vi "Boiler room teest 2.vi"() -> ()   [LabVIEW 2023]
uses:
  Heater.vi
  AC.vi
panel:
  out "temp":dbl
  in  "?":dbl(knob) min=0.0 max=2.0 step=1.0 scale=0.0..2.0
  in  "stop":bool
  out "Thermometer":dbl(slide) scale=0.0..100.0
  in  "min temp":dbl=20.0
  in  "max temp":dbl=80.0
  in  "Automatic / Manual":bool
  out "AC":bool
  out "Heater":bool
  # "Heater"
  # "OFF"
  # "AC"
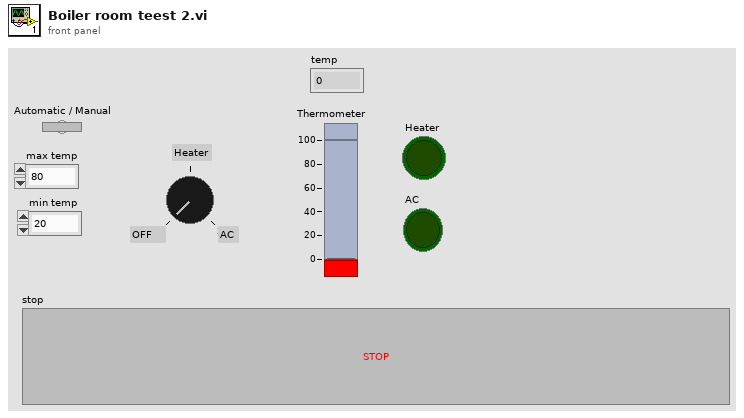
[diagram p1: front panel]
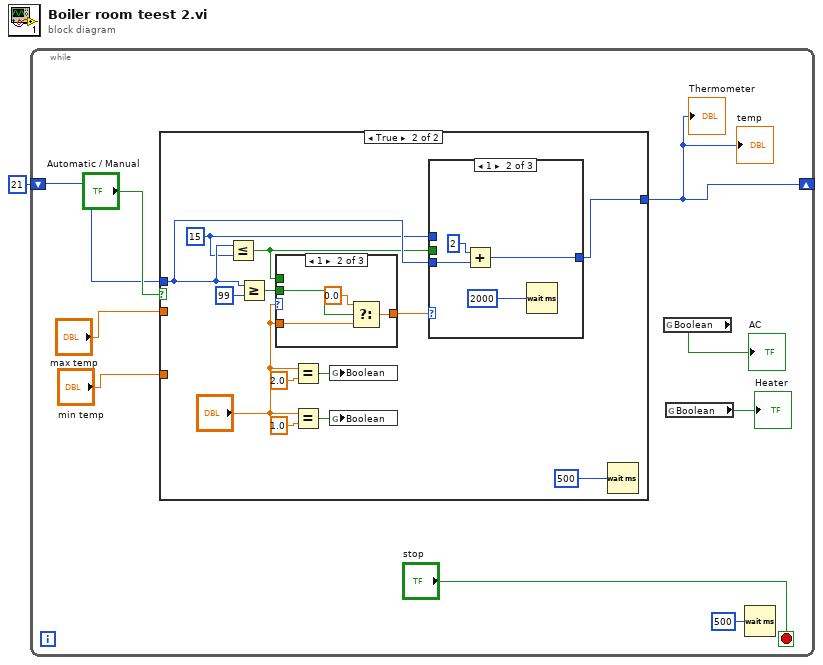
[diagram p0: block diagram]
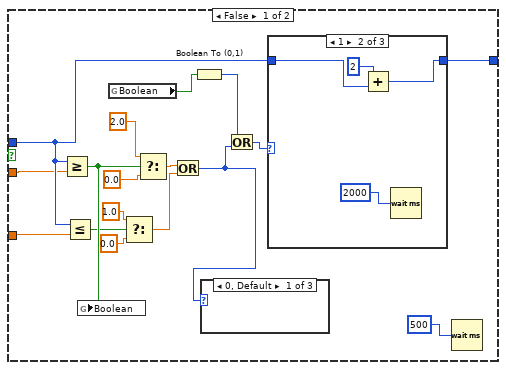
[diagram p2: hidden frame]
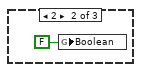
[diagram p3: hidden frame]
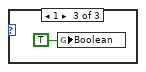
[diagram p4: hidden frame]
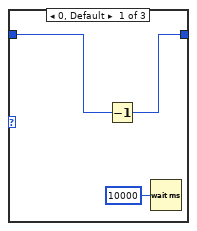
[diagram p5: hidden frame]
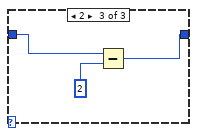
[diagram p6: hidden frame]
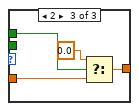
[diagram p8: hidden frame]
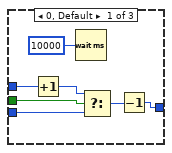
[diagram p9: hidden frame]
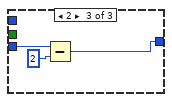
[diagram p10: hidden frame]
diagram:
  n1 = while {
    shift-right: [w5] -> _
    shift-left: 21 -> [w2]
    stop <- "stop" stop-if-true
    n2 = case shown="True" "Automatic / Manual" {
      tunnel: w2 -> [w20 w45]
      tunnel: "max temp" -> [w19 _]
      tunnel: "min temp" -> [w18 _]
      tunnel: [w22 w51] -> w5
      frame False {
        n3 = Greater Or Equal?(x=w20, y=w19) -> (x >= y?=w16:bool)
        n4 = Less Or Equal?(x=w20, y=w18) -> (x <= y?=w15:bool)
        n5 = global write "AC.vi" "Boolean"(w16) -> ()
        n6 = global read "Heater.vi" "Boolean"() -> (w11:bool)
        n7 = Select(t=1.0, s=w15, f=0.0) -> (s? t:f=w17:dbl)
        n8 = Select(t=2.0, s=w16, f=0.0) -> (s? t:f=w23:dbl)
        n9 = Or(x=w23, y=w17) -> (x .or. y?=w14:i32)
        n10 = Boolean To (0,1)(Boolean=w11) -> (0, 1=w12:i16)
        n11 = case shown="0, Default" w14 {
          frame 0, Default {
          }
          frame 2 {
            n12 = global write "Heater.vi" "Boolean"(FALSE ("Boolean")) -> ()
          }
          frame 1 {
            n13 = global write "Heater.vi" "Boolean"(TRUE ("Boolean")) -> ()
          }
        }
        n14 = Or(x=w12, y=w14) -> (x .or. y?=w13:i32)
        n15 = case shown="1" w13 {
          tunnel: w20 -> [w32 w36 w39]
          tunnel: [w31 w34 w38] -> w22
          frame 0, Default {
            n16 = Decrement(x=w32) -> (x-1=w31:i32)
            n17 = Wait (ms)(milliseconds to wait=u32 10000) -> ()  [unwired: 1 out]
          }
          frame 1 {
            n18 = Add(x=2, y=w36) -> (x+y=w34:i32)
            n19 = Wait (ms)(milliseconds to wait=u32 2000) -> ()  [unwired: 1 out]
          }
          frame 2 {
            n20 = Subtract(x=w39, y=2) -> (x-y=w38:i32)
          }
        }
        n21 = Wait (ms)(milliseconds to wait=u32 500) -> ()  [unwired: 1 out]
      }
      frame True {
        w40 = 15
        n22 = Less Or Equal?(x=w45, y=w40) -> (x <= y?=w41:bool)
        n23 = Greater Or Equal?(x=w45, y=99 ("x")) -> (x >= y?=w42:bool)
        n24 = case shown="1" "?" {
          tunnel: "?" -> [w53 w54 w59]
          tunnel: [w53 w56 w60] -> w50
          tunnel: w42 -> [_ w57 _]
          tunnel: w41 -> [_ _ w61]
          frame 0, Default {
          }
          frame 1 {
            n25 = Select(t=0.0 ("f"), s=w57, f=w54) -> (s? t:f=w56:dbl)
          }
          frame 2 {
            n26 = Select(t=0.0, s=w61, f=w59) -> (s? t:f=w60:dbl)
          }
        }
        n27 = Equal?(x="?", y=2.0) -> (x = y?=w46:bool)
        n28 = Equal?(x="?", y=1.0) -> (x = y?=w48:bool)
        n29 = global write "AC.vi" "Boolean"(w46) -> ()
        n30 = global write "Heater.vi" "Boolean"(w48) -> ()
        n31 = case shown="1" w50 {
          tunnel: w45 -> [w65 w72 w75]
          tunnel: [w68 w71 w74] -> w51
          tunnel: w41 -> [w66 _ _]
          tunnel: w40 -> [w63 _ _]
          frame 0, Default {
            n32 = Increment(x=w63) -> (x+1=w62:i32)
            n33 = Wait (ms)(milliseconds to wait=u32 10000) -> ()  [unwired: 1 out]
            n34 = Select(t=w62, s=w66, f=w65) -> (s? t:f=w64:i32)
            n35 = Decrement(x=w64) -> (x-1=w68:i32)
          }
          frame 1 {
            n36 = Add(x=2, y=w72) -> (x+y=w71:i32)
            n37 = Wait (ms)(milliseconds to wait=u32 2000) -> ()  [unwired: 1 out]
          }
          frame 2 {
            n38 = Subtract(x=w75, y=2) -> (x-y=w74:i32)
          }
        }
        n39 = Wait (ms)(milliseconds to wait=u32 500) -> ()  [unwired: 1 out]
      }
    }
    "Thermometer" <- w5
    "temp" <- w5
    n40 = global read "AC.vi" "Boolean"() -> (→"AC":bool)
    n41 = global read "Heater.vi" "Boolean"() -> (→"Heater":bool)
    n42 = Wait (ms)(milliseconds to wait=u32 500) -> ()  [unwired: 1 out]
  }
